vi "Multi Boolean F-I Test.vi"() -> ()   [LabVIEW 2021]
uses:
  Source/Omni-Bus/Omni_Bus.lvclass
  Source/Omni-Bus/Support/Broad Types.ctl
  Source/Local Bus/Local Bus.lvclass
  C:/Users/Tim/Documents/GitHub/Omni-Bus/Source/Omni-Bus/Bus Access/Bus_Access.lvclass
  <vilib>/Utility/Data Type/Type Definitions/Data Type.ctl
  Source/Fault-Injection Bus/Fault-Injection Bus.lvclass
  <vilib>/TSA/Abstract Data Classes/Abs_Types/Type/Abs_Type.lvclass/Abs_Type.ctl
  Source/Omni-Bus/Omni_Bus.lvclass/Omni_Bus.ctl
  Source/Omni-Bus/Support/FindVar.vi
  Source/Omni-Bus/Support/Get/Get Multi Boolean.vi
  <vilib>/Utility/error.llb/Clear Errors.vi
  Source/Omni-Bus/Properties/Read Var Map.vi
  <vilib>/TSA/Abstract Data Classes/Abs_Types/Type/Properties/Read Tag.vi
  Source/Omni-Bus/Support/FindMultiVar.vi
  <vilib>/TSA/Abstract Data Classes/Abs_Types/Boolean/Abs_Boolean.lvclass
  C:/Program Files (x86)/National Instruments/LabVIEW 2021/vi.lib/TSA/Abstract Data Classes/Abs_Types/Type/Abs_Type.lvclass
  <vilib>/TSA/Abstract Data Classes/Abs_Types/Value/Abs_Value.lvclass
  Source/Omni-Bus/Support/Check For Read Only Error.vi
  Source/Omni-Bus/Support/Incorrect Tag String Error.vi
  <vilib>/TSA/Abstract Data Classes/Abs_Types/Type/Abs_Type.lvclass
  <vilib>/Utility/Data Type/NI_Data Type.lvlib
  C:/Users/Tim/Documents/GitHub/Omni-Bus/Source/Local Bus/Local Bus.lvclass
  C:/Users/Tim/Documents/GitHub/Omni-Bus/Source/Fault-Injection Bus/Fault-Injection Bus.lvclass
panel:
  in  "Enable":bool[](array[boolean])
  in  "Injected Value":bool[](array[boolean])
  in  "Tag 4":string[](array[combo])
  out "error out 4":errorcluster
  in  "Arm":bool
  in  "Array":bool[](array[boolean])
  out "Booleans":bool[](array[boolean])
  out "error out 3":errorcluster
  out "error out 2":errorcluster
  in  "Tag 2":string[](array[combo])
  in  "stop":bool
  in  "Tags":string[](array[combo])
  out "error out":errorcluster
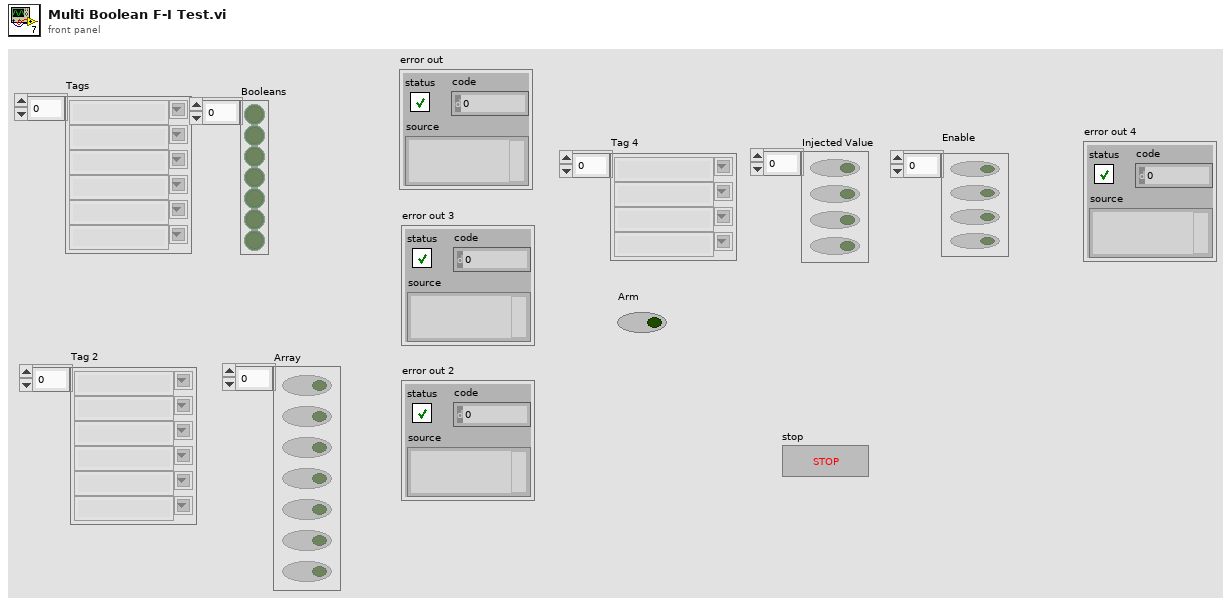
[diagram p1: front panel]
types:
  T1 = typedef "NI_Data Type.lvlib/Data Type.ctl" = enum8{"Invalid Type", "Void", "I8", "I16", "I32", "I64", "U8", "U16", "U32", "U64", "Single Float", "Double Float", "Extended Float", "Single Complex", "Double Complex", "Extended Complex", "Enum U8", "Enum U16", "Enum U32", "Enum U64", "Single Float With Unit", "Double Float With Unit", "Extended Float With Unit", "Single Complex with Unit", "Double Complex with Unit", "Extended Complex with Unit", "Boolean", "String", "Path", "Picture", "Tag", "Array", "Cluster", "Variant", "LV Variant", "Waveform", "Timestamp", "Digital Waveform", "Digital Data", "ExpressData", "Refnum", "External Data", "VI", "Poly VI", "LabVIEW Class Instance", "Fixed Point", "Set Collection", "Map Collection"}
  T2 = typedef "Omni_Bus.lvclass/Broad Types.ctl" = enum16{"All Tags", "NI Specific Type", "Boolean", "String", "Numeric", "Float", "Integer", "Collection", "All Value Types", "Non Value Types"}
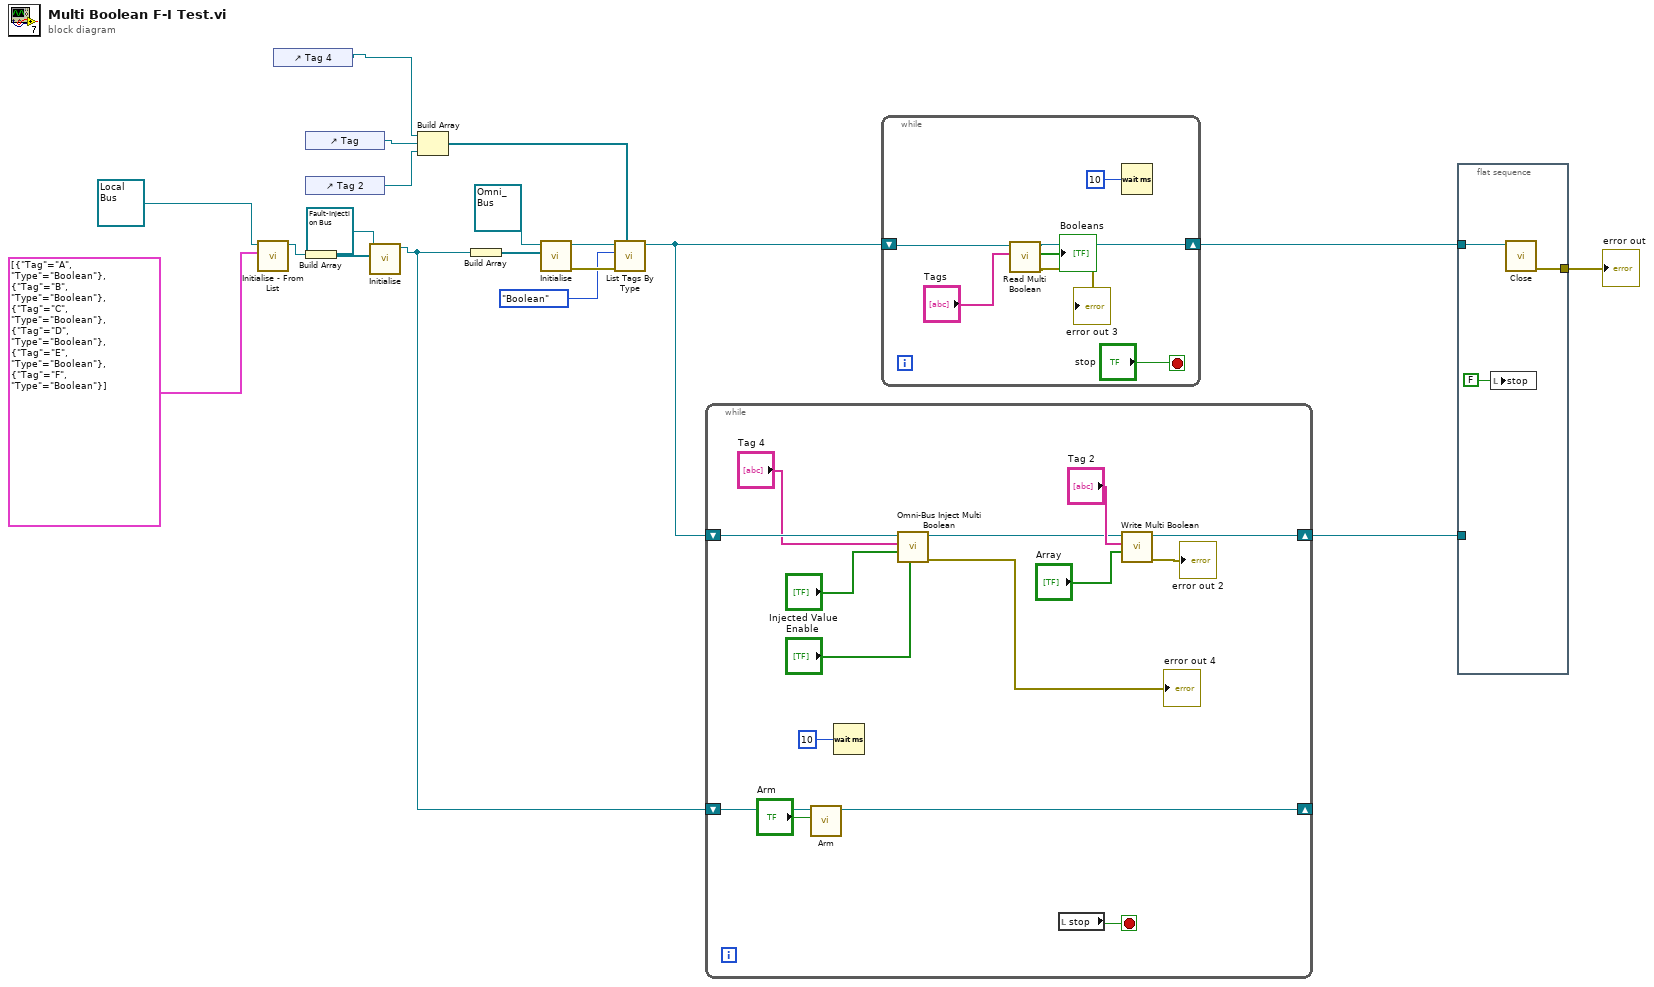
[diagram p0: block diagram]
diagram:
  n1 = call "Initialise - From List.vi"("Tag List"=cluster{"Tag":string, "Type":T1}[] [{"Tag"="A", "Type"=enum."Boolean"}, {"Tag"="B", "Type"=enum."Boolean"}, {"Tag"="C", "Type"=enum."Boolean"}, {"Tag"="D", "Type"=enum."Boolean"}, {"Tag"="E", "Type"=enum."Boolean"}, {"Tag"="F", "Type"=enum."Boolean"}], "Local Bus in"=refnum<class "Local Bus.lvclass"> refnum ("Local Bus.lvclass")) -> ("Local Bus out"=w5:refnum<class "Local Bus.lvclass">)  [unwired: 8 in, 1 out]
  n2 = control-ref of="Tag 4"() -> (w1:refnum<vi>)
  n3 = control-ref of="Tag"() -> (w8:refnum<vi>)
  n4 = control-ref of="Tag 2"() -> (w7:refnum<vi>)
  n5 = Build Array(w5) -> (w4:refnum<class "Local Bus.lvclass">[])
  n6 = call "Initialise.vi"("Buses"=w4, "Fault-Injection Bus in"=refnum<class "Fault-Injection Bus.lvclass"> refnum) -> ("Fault-Injection Bus out"=w2:refnum<class "Fault-Injection Bus.lvclass">)  [unwired: 8 in, 1 out]
  n7 = Build Array(w1, w8, w7) -> (w6:refnum<vi>[])
  n8 = Build Array(w2) -> (w18:refnum<class "Fault-Injection Bus.lvclass">[])
  n9 = call-dynamic "Initialise.vi"("Bus Access"=w18, "Var Bus in"=refnum<class "Omni_Bus.lvclass"> refnum) -> ("error out"=w16:errorcluster, "Var Bus out"=w17:refnum<class "Omni_Bus.lvclass">)  [unwired: 8 in]
  n10 = call "List Tags By Type.vi"("Combo Boxes"=w6, "error in (no error)"=w16, "Broad Types"=Broad_Types."Boolean", "Var Bus in"=w17) -> ("Var Bus out"=w12:refnum<class "Omni_Bus.lvclass">)  [unwired: 4 in, 3 out]
  n11 = while {
    shift-right: [w32] -> w11
    shift-left: w12 -> [w25]
    shift-right: [w26] -> _
    shift-left: w2 -> [w28]
    stop <- w34 stop-if-true
    n12 = call "Arm.vi"("Arm"="Arm", "Fault-Injection Bus in"=w28) -> ("Fault-Injection Bus out"=w26:refnum<class "Fault-Injection Bus.lvclass">)  [unwired: 8 in, 1 out]
    n13 = Wait (ms)(milliseconds to wait=u32 10) -> ()  [unwired: 1 out]
    n14 = call "Omni-Bus Inject Multi Boolean.vi"("Enable"="Enable", "Injected Values"="Injected Value", "Tag"="Tag 4", "Omni_Bus in"=w25) -> ("error out"=→"error out 4":errorcluster, "Omni_Bus out"=w24:refnum<class "Omni_Bus.lvclass">)  [unwired: 6 in]
    n15 = local read "stop"() -> (w34:bool)
    n16 = call "Write Multi Boolean.vi"("Array"="Array", "Tag"="Tag 2", "Omni_Bus in"=w24) -> ("error out"=→"error out 2":errorcluster, "Omni_Bus out"=w32:refnum<class "Omni_Bus.lvclass">)  [unwired: 7 in]
  }
  n17 = while {
    shift-right: [w39] -> w13
    shift-left: w12 -> [w38]
    stop <- "stop" stop-if-true
    n18 = call "Read Multi Boolean.vi"("Tags"="Tags", "Var Bus in"=w38) -> ("error out"=→"error out 3":errorcluster, "Booleans"=→"Booleans":bool[], "Var Bus out"=w39:refnum<class "Omni_Bus.lvclass">)  [unwired: 7 in]
    n19 = Wait (ms)(milliseconds to wait=u32 10) -> ()  [unwired: 1 out]
  }
  n20 = flat-sequence {
    tunnel: [w44] -> w14
    tunnel: w13 -> [w43]
    tunnel: w11 -> [_]
    frame #0 {
      n21 = local write "stop"(FALSE ("stop")) -> ()
      n22 = call-dynamic "Close.vi"("Data in"=w43) -> ("error out"=w44:errorcluster)  [unwired: 9 in, 1 out]
    }
  }
  "error out" <- w14
